vi "Process.vi"(11 "error in":errorcluster) -> (3 "error out":errorcluster)   [LabVIEW 2015]
uses:
  Controls/Global Vairable.vi
panel:
  # "Please wait....."
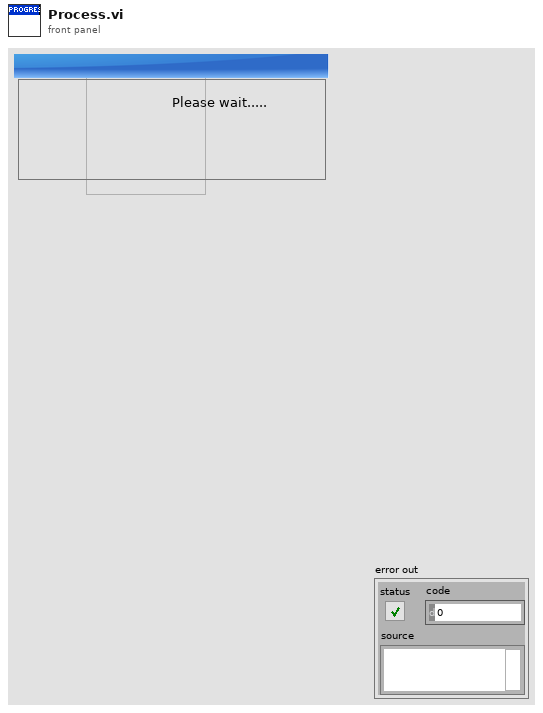
[diagram p1: front panel]
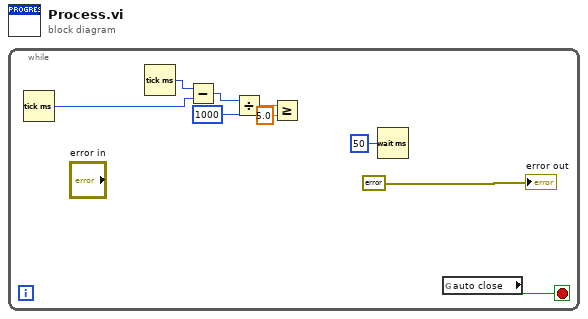
[diagram p0: block diagram]
diagram:
  n1 = while {
    stop <- w2 stop-if-true
    n2 = Tick Count (ms)() -> (millisecond timer value=w9:u32)
    n3 = Tick Count (ms)() -> (millisecond timer value=w7:u32)
    n4 = Subtract(x=w7, y=w9) -> (x-y=w6:u32)
    n5 = Divide(x=w6, y=u32 1000) -> (x/y=w4:dbl)
    n6 = Greater Or Equal?(x=w4, y=5.0) -> ()  [unwired: 1 out]
    n7 = Wait (ms)(milliseconds to wait=u32 50) -> ()  [unwired: 1 out]
    n8 = global read "Global Vairable.vi" "auto close"() -> (w2:bool)
    "error out" <- errorcluster {"status"=FALSE, "code"=0, "source"=""} ("error out")
  }
